vi "TwithFPOStarterCode.vi"() -> ()   [LabVIEW 2019]
doc: "EE 200 Problem Set 7 Problem 25"
uses:
  Downloads/Project 2/Project 2/state.ctl
panel:
  out "Thermostat Signal":u32[](array[colorbox])
  in  "Reset":bool
  out "Clock":bool
  out "Present State":T1
  out "Clock Cycle":i32
  in  "Sensors":bool[](array[boolean])
  in  "Stop Button":bool
  # "Thermostat"
  # "H\n\nC\n\nB"
  # "Standby \n\n\nCharging\n\n\nCooling\n\n\nHeating"
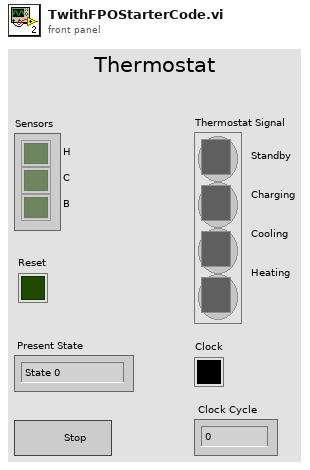
[diagram p1: front panel]
types:
  T1 = typedef "state.ctl" = enum16{"State 0", "State 1", "State 2", "State 3"}
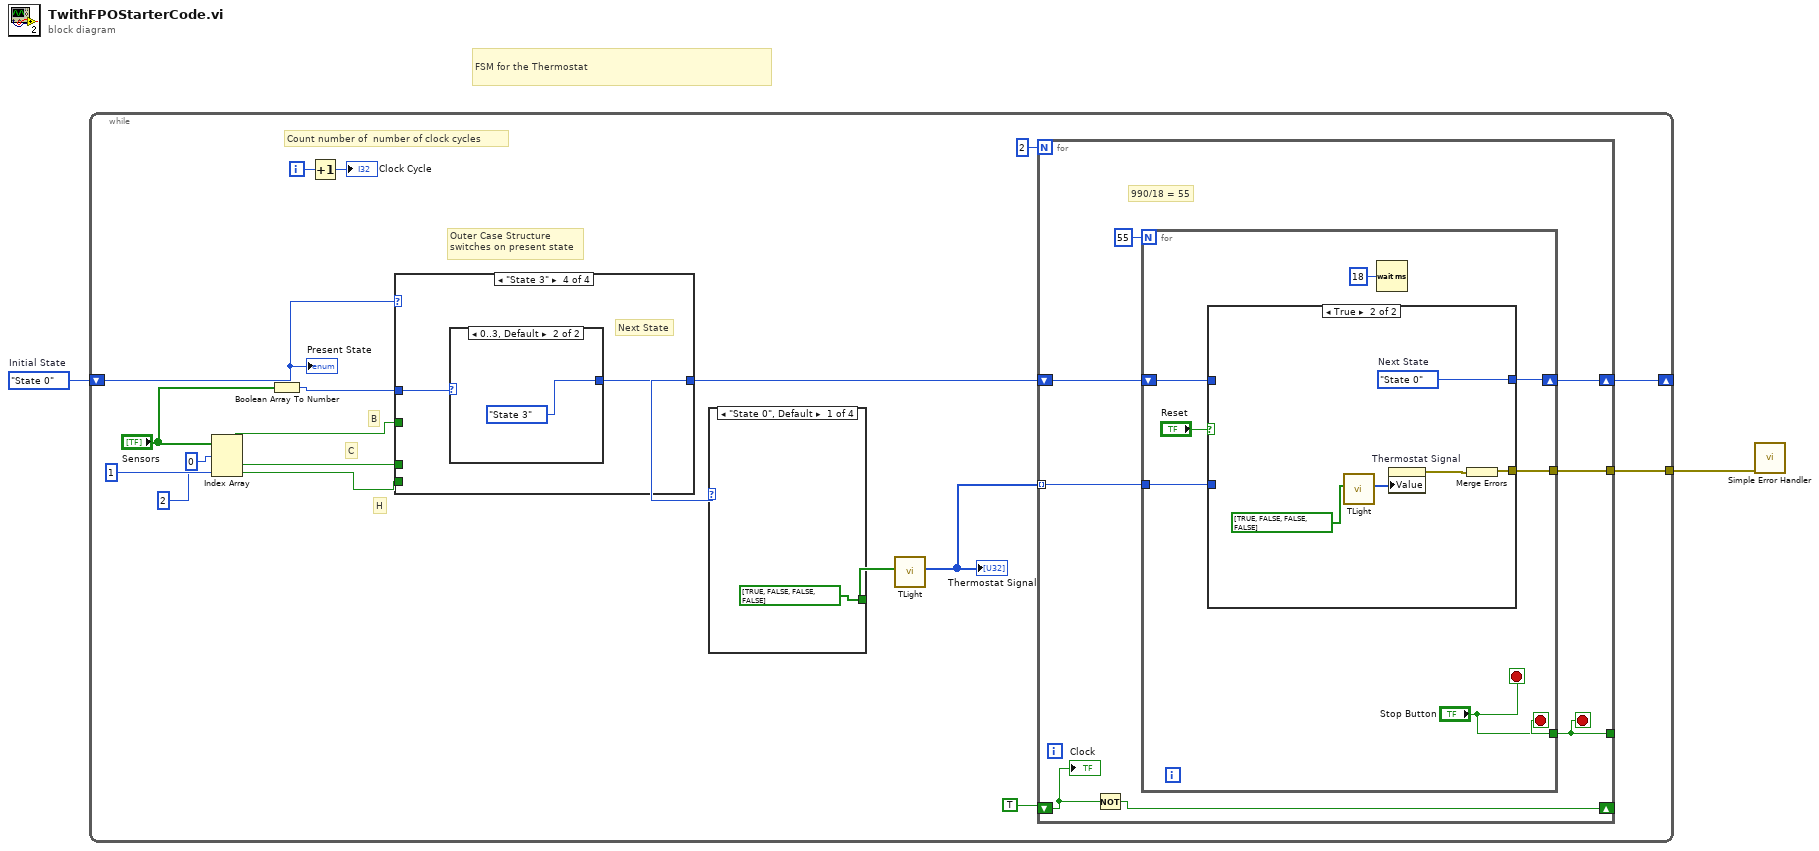
[diagram p0: block diagram]
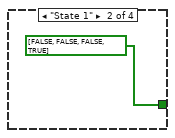
[diagram p2: hidden frame]
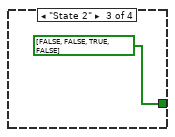
[diagram p3: hidden frame]
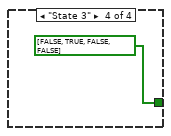
[diagram p4: hidden frame]
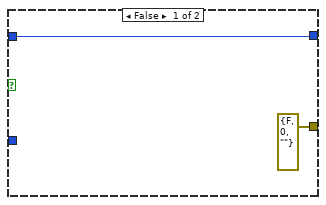
[diagram p5: hidden frame]
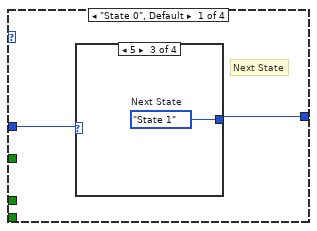
[diagram p6: hidden frame]
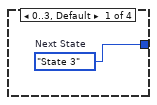
[diagram p7: hidden frame]
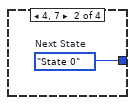
[diagram p8: hidden frame]
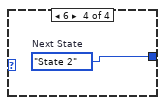
[diagram p9: hidden frame]
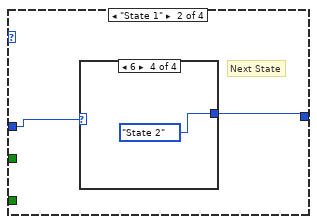
[diagram p10: hidden frame]
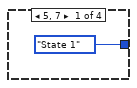
[diagram p11: hidden frame]
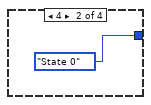
[diagram p12: hidden frame]
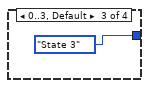
[diagram p13: hidden frame]
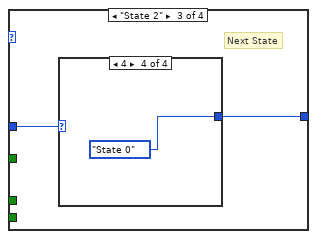
[diagram p14: hidden frame]
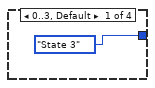
[diagram p15: hidden frame]
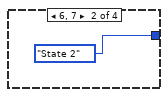
[diagram p16: hidden frame]
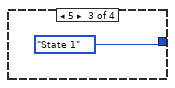
[diagram p17: hidden frame]
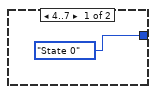
[diagram p18: hidden frame]
diagram:
  w2 = state."State 0"  # Initial State
  # "FSM for the Thermostat"
  n1 = while {
    shift-right: [w16] -> _
    shift-left: w2 -> [w19]
    tunnel: [w14] -> w1
    i -> [w21]
    stop <- w18 stop-if-true
    # "H"
    # "C"
    # "B"
    # "Count number of  number of clock cycles"
    # "Outer Case Structure \nswitches on present state"
    n2 = Index Array(array="Sensors", index #1=0 ("index"), index #2=1 ("index"), index #3=2 ("index")) -> (element #1=w5:bool, element #2=w4:bool, element #3=w3:bool)
    n3 = Boolean Array To Number(Boolean array="Sensors") -> (number=w9:u32)
    n4 = Increment(x=w21) -> (x+1=→"Clock Cycle":i32)
    n5 = case shown="\"State 3\"" w19 {
      tunnel: [w49 w55 w61 w67] -> w15
      tunnel: w9 -> [w48 w54 w60 w66]
      tunnel: w5 -> [_ _ _ _]
      tunnel: w4 -> [_ _ _ _]
      tunnel: w3 -> [_ _ _ _]
      frame "State 0", Default {
        # "Next State"
        n6 = case shown="5" w48 {
          tunnel: [w50 w51 w52 w53] -> w49
          frame 0..3, Default {
            w50 = state."State 3"  # Next State
          }
          frame 4, 7 {
            w51 = state."State 0"  # Next State
          }
          frame 5 {
            w52 = state."State 1"  # Next State
          }
          frame 6 {
            w53 = state."State 2"  # Next State
          }
        }
      }
      frame "State 1" {
        # "Next State"
        n7 = case shown="6" w54 {
          tunnel: [state."State 1" ("Present State") state."State 0" ("Present State") state."State 3" ("Present State") state."State 2" ("Present State")] -> w55
          frame 5, 7 {
          }
          frame 4 {
          }
          frame 0..3, Default {
          }
          frame 6 {
          }
        }
      }
      frame "State 2" {
        # "Next State"
        n8 = case shown="4" w60 {
          tunnel: [state."State 3" ("Present State") state."State 2" ("Present State") state."State 1" ("Present State") state."State 0" ("Present State")] -> w61
          frame 0..3, Default {
          }
          frame 6, 7 {
          }
          frame 5 {
          }
          frame 4 {
          }
        }
      }
      frame "State 3" {
        # "Next State"
        n9 = case shown="0..3, Default" w66 {
          tunnel: [state."State 0" ("Present State") state."State 3" ("Present State")] -> w67
          frame 4..7 {
          }
          frame 0..3, Default {
          }
        }
      }
    }
    n10 = case shown="\"State 0\", Default" w15 {
      tunnel: [bool[] [TRUE, FALSE, FALSE, FALSE] bool[] [FALSE, FALSE, FALSE, TRUE] bool[] [FALSE, FALSE, TRUE, FALSE] bool[] [FALSE, TRUE, FALSE, FALSE]] -> w13
      frame "State 0", Default {
      }
      frame "State 1" {
      }
      frame "State 2" {
      }
      frame "State 3" {
      }
    }
    n11 = call "TLight.vi"("Array"=w13) -> ("Array 2"=w12:u32[])  [unwired: 10 in]
    "Thermostat Signal" <- w12
    n12 = for {
      N: 2 -> [_]
      shift-right: [w31] -> w16
      shift-left: w15 -> [w32]
      tunnel: [w33] -> w18
      shift-right: [w28] -> _
      shift-left: TRUE -> [w29]
      tunnel: [w30] -> w14
      tunnel: w12 -> [w27] mode=indexing
      stop <- w33 stop-if-true
      # "990/18 = 55"
      n13 = Not(x=w29) -> (.not. x?=w28:bool)
      n14 = for {
        N: 55 -> [_]
        tunnel: ["Stop Button"] -> w33
        shift-right: [w39] -> w31
        shift-left: w32 -> [w38]
        tunnel: [w36] -> w30
        tunnel: w27 -> [w35]
        stop <- "Stop Button" stop-if-true
        n15 = case shown="True" "Reset" {
          tunnel: [w42 w47] -> w39
          tunnel: w38 -> [w42 _]
          tunnel: [errorcluster {"status"=FALSE, "code"=0, "source"=""} ("error constant") w46] -> w36
          tunnel: w35 -> [_ _]
          frame False {
          }
          frame True {
            w47 = state."State 0"  # Next State
            n16 = call "TLight.vi"("Array"=bool[] [TRUE, FALSE, FALSE, FALSE]) -> ("Array 2"=w43:u32[])  [unwired: 10 in]
            n17 = property on="Thermostat Signal" class="Arr (strict)"("Value"=w43) -> (error out=w45:errorcluster)  [unwired: 2 in, 1 out]
            n18 = Merge Errors(w45) -> (w46:errorcluster)
          }
        }
        n19 = Wait (ms)(milliseconds to wait=u32 18) -> ()  [unwired: 1 out]
      }
      "Clock" <- w29
    }
    "Present State" <- w19
  }
  n20 = call <vilib>:"Simple Error Handler.vi"("error in (no error)"=w1) -> ()  [unwired: 4 in, 5 out]
